vi "XY Graph Number of Plots.vi"(8 "Error In":errorcluster, 11 "XYGraph in":T1) -> (0 "Error Out":errorcluster, 3 "# Plots":i32)   [LabVIEW 2019]
uses:
  XY Graph Refnum.ctl
  XY Graph Add-Ons.lvlib
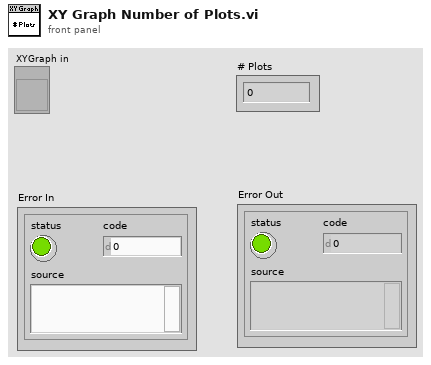
[diagram p1: front panel]
types:
  T1 = typedef "XY Graph Add-Ons.lvlib/XY Graph Refnum.ctl" = refnum<vi>
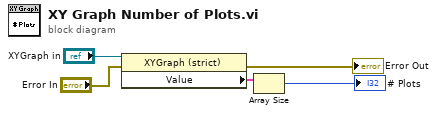
[diagram p0: block diagram]
diagram:
  n1 = property class="XYGraph (strict)"(reference="XYGraph in", error in="Error In") -> (error out=→"Error Out":errorcluster, "Value"=w2:cluster{"X Array":dbl[], "Y Array":dbl[]}[])  [unwired: 1 out]
  n2 = Array Size(array=w2) -> (size(s)=→"# Plots":i32)
